vi "test Init Anaylsis Graph 1.vi"(11 "Test Case In":refnum<class "test Init Analysis Graph.lvclass">) -> (0 "error out":errorcluster, 3 "Test Case Out":refnum<class "test Init Analysis Graph.lvclass">)   [LabVIEW 2023, in "test Init Analysis Graph.lvclass"]
uses:
  test Init Analysis Graph.lvclass
  C:/Program Files/National Instruments/LabVIEW 2023/vi.lib/Astemes/LUnit/Test Case.lvclass
  source/Base Graph/Base Graph.lvclass/Base Graph.ctl
  source/Series Graph/Graph with Series View.lvclass/Graph with Series View.ctl
  source/Analysis Graph/Graph with Analysis Controls.lvclass/Graph with Analysis Controls.ctl
  <vilib>/Astemes/LUnit/Test Case.lvclass/Test Case.ctl
  source/Base Graph/Get Cursor Position.vi
  source/Series Graph/Get 1D Array Image Index and Length.vi
  source/Base Graph/Get Size.vi
  source/Series Graph/Get Shots.vi
  source/Analysis Graph/Update Z Cursors.vi
  <vilib>/Astemes/LUnit/Append Pass Result.vi
  <vilib>/Astemes/LUnit/Append Fail Result.vi
  source/Analysis Graph/Get Analysis ROI.vi
  source/Series Graph/Get Series Graph.vi
  <vilib>/Astemes/LUnit/Run In UI.vi
  source/Base Graph/Get ROI X-Y.vi
  <vilib>/Utility/error.llb/Clear Errors.vi
  source/Analysis Graph/Graph with Analysis Controls.lvclass
  D:/git/Lock-In-Thermography-Graphs/source/Series Graph/Graph with Series View.lvclass
  D:/git/Lock-In-Thermography-Graphs/source/Base Graph/Base Graph.lvclass
  source/Series Graph/Graph with Series View.lvclass
  <vilib>/Astemes/LUnit/Test Case.lvclass
  <vilib>/Analysis/NI_AALBase.lvlib
panel:
  in  "Z Range":cluster{"Index":u32, "Length":u32}={"Index"=0, "Length"=999}
  out "Signal Map Analysis":dbl[][](graph)
  out "Intensity Height Graph Analysis":cluster{"Array":dbl[], "Array":dbl[]}(graph)={"Array"=array[480 elements], "Array"=[0.0, 1.0, 2.0, 3.0, 4.0, 5.0, 6.0, 7.0, 8.0, 9.0, 10.0, 11.0, 12.0, 13.0, 14.0, 15.0, 16.0, 17.0, 18.0, 19.0, 20.0, 21.0, 22.0, 23.0, 24.0, 25.0, 26.0, 27.0, 28.0, 29.0, 30.0, 31.0, 32.0, 33.0, 34.0, 35.0, 36.0, 37.0, 38.0, 39.0, 40.0, 41.0, 42.0, 43.0, 44.0, 45.0, 46.0, 47.0, 48.0, 49.0, 50.0, 51.0, 52.0, 53.0, 54.0, 55.0, 56.0, 57.0, 58.0, 59.0, 60.0, 61.0, 62.0, 63.0, 64.0, 65.0, 66.0, 67.0, 68.0, 69.0, 70.0, 71.0, 72.0, 73.0, 74.0, 75.0, 76.0, 77.0, 78.0, 79.0, 80.0, 81.0, 82.0, 83.0, 84.0, 85.0, 86.0, 87.0, 88.0, 89.0, 90.0, 91.0, 92.0, 93.0, 94.0, 95.0, 96.0, 97.0, 98.0, 99.0, 100.0, 101.0, 102.0, 103.0, 104.0, 105.0, 106.0, 107.0, 108.0, 109.0, 110.0, 111.0, 112.0, 113.0, 114.0, 115.0, 116.0, 117.0, 118.0, 119.0, 120.0, 121.0, 122.0, 123.0, 124.0, 125.0, 126.0, 127.0, 128.0, 129.0, 130.0, 131.0, 132.0, 133.0, 134.0, 135.0, 136.0, 137.0, 138.0, 139.0, 140.0, 141.0, 142.0, 143.0, 144.0, 145.0, 146.0, 147.0, 148.0, 149.0, 150.0, 151.0, 152.0, 153.0, 154.0, 155.0, 156.0, 157.0, 158.0, 159.0, 160.0, 161.0, 162.0, 163.0, 164.0, 165.0, 166.0, 167.0, 168.0, 169.0, 170.0, 171.0, 172.0, 173.0, 174.0, 175.0, 176.0, 177.0, 178.0, 179.0, 180.0, 181.0, 182.0, 183.0, 184.0, 185.0, 186.0, 187.0, 188.0, 189.0, 190.0, 191.0, 192.0, 193.0, 194.0, 195.0, 196.0, 197.0, 198.0, 199.0, 200.0, 201.0, 202.0, 203.0, 204.0, 205.0, 206.0, 207.0, 208.0, 209.0, 210.0, 211.0, 212.0, 213.0, 214.0, 215.0, 216.0, 217.0, 218.0, 219.0, 220.0, 221.0, 222.0, 223.0, 224.0, 225.0, 226.0, 227.0, 228.0, 229.0, 230.0, 231.0, 232.0, 233.0, 234.0, 235.0, 236.0, 237.0, 238.0, 239.0, 240.0, 241.0, 242.0, 243.0, 244.0, 245.0, 246.0, 247.0, 248.0, 249.0, 250.0, 251.0, 252.0, 253.0, 254.0, 255.0, 256.0, 257.0, 258.0, 259.0, 260.0, 261.0, 262.0, 263.0, 264.0, 265.0, 266.0, 267.0, 268.0, 269.0, 270.0, 271.0, 272.0, 273.0, 274.0, 275.0, 276.0, 277.0, 278.0, 279.0, 280.0, 281.0, 282.0, 283.0, 284.0, 285.0, 286.0, 287.0, 288.0, 289.0, 290.0, 291.0, 292.0, 293.0, 294.0, 295.0, 296.0, 297.0, 298.0, 299.0, 300.0, 301.0, 302.0, 303.0, 304.0, 305.0, 306.0, 307.0, 308.0, 309.0, 310.0, 311.0, 312.0, 313.0, 314.0, 315.0, 316.0, 317.0, 318.0, 319.0, 320.0, 321.0, 322.0, 323.0, 324.0, 325.0, 326.0, 327.0, 328.0, 329.0, 330.0, 331.0, 332.0, 333.0, 334.0, 335.0, 336.0, 337.0, 338.0, 339.0, 340.0, 341.0, 342.0, 343.0, 344.0, 345.0, 346.0, 347.0, 348.0, 349.0, 350.0, 351.0, 352.0, 353.0, 354.0, 355.0, 356.0, 357.0, 358.0, 359.0, 360.0, 361.0, 362.0, 363.0, 364.0, 365.0, 366.0, 367.0, 368.0, 369.0, 370.0, 371.0, 372.0, 373.0, 374.0, 375.0, 376.0, 377.0, 378.0, 379.0, 380.0, 381.0, 382.0, 383.0, 384.0, 385.0, 386.0, 387.0, 388.0, 389.0, 390.0, 391.0, 392.0, 393.0, 394.0, 395.0, 396.0, 397.0, 398.0, 399.0, 400.0, 401.0, 402.0, 403.0, 404.0, 405.0, 406.0, 407.0, 408.0, 409.0, 410.0, 411.0, 412.0, 413.0, 414.0, 415.0, 416.0, 417.0, 418.0, 419.0, 420.0, 421.0, 422.0, 423.0, 424.0, 425.0, 426.0, 427.0, 428.0, 429.0, 430.0, 431.0, 432.0, 433.0, 434.0, 435.0, 436.0, 437.0, 438.0, 439.0, 440.0, 441.0, 442.0, 443.0, 444.0, 445.0, 446.0, 447.0, 448.0, 449.0, 450.0, 451.0, 452.0, 453.0, 454.0, 455.0, 456.0, 457.0, 458.0, 459.0, 460.0, 461.0, 462.0, 463.0, 464.0, 465.0, 466.0, 467.0, 468.0, 469.0, 470.0, 471.0, 472.0, 473.0, 474.0, 475.0, 476.0, 477.0, 478.0, 479.0]}
  out "Intensity Width Graph Analysis":cluster{"Array":dbl[], "Array":dbl[]}(graph)
  out "Z - Time Signal":u16[](graph)=[8685, 8675, 8685, 8678, 8689, 8675, 8659, 8679, 8685, 8681, 8681, 8682, 8675, 8687, 8678, 8679, 8686, 8681, 8671, 8674, 8685, 8680, 8679, 8667, 8687, 8682, 8683, 8675, 8675, 8677, 8683, 8679, 8685, 8686, 8687, 8679, 8688, 8683, 8679, 8683, 8681, 8685, 8684, 8677, 8677, 8680, 8677, 8674, 8697, 8693, 8683, 8704, 8687, 8692, 8700, 8688, 8691, 8687, 8699, 8697, 8693, 8710, 8707, 8709, 8693, 8711, 8690, 8699, 8699, 8710, 8709, 8700, 8712, 8701, 8714, 8718, 8710, 8723, 8717, 8718, 8727, 8731, 8715, 8724, 8729, 8735, 8725, 8745, 8724, 8730, 8746, 8744, 8740, 8729, 8737, 8722, 8748, 8727, 8736, 8747, 8746, 8742, 8739, 8752, 8746, 8745, 8748, 8748, 8738, 8737, 8737, 8747, 8770, 8768, 8766, 8763, 8774, 8769, 8761, 8753, 8758, 8747, 8766, 8775, 8780, 8771, 8775, 8785, 8766, 8778, 8762, 8772, 8783, 8785, 8778, 8778, 8787, 8796, 8807, 8798, 8789, 8792, 8804, 8799, 8794, 8799, 8796, 8805, 8789, 8792, 8805, 8813, 8805, 8796, 8805, 8798, 8812, 8816, 8811, 8809, 8821, 8821, 8808, 8804, 8818, 8822, 8826, 8829, 8810, 8834, 8808, 8820, 8814, 8821, 8822, 8825, 8825, 8830, 8836, 8821, 8842, 8826, 8819, 8820, 8841, 8827, 8833, 8838, 8835, 8842, 8830, 8839, 8829, 8831, 8839, 8849, 8838, 8842, 8836, 8844, 8832, 8845, 8841, 8857, 8858, 8844, 8836, 8839, 8828, 8856, 8843, 8854, 8851, 8852, 8837, 8827, 8848, 8864, 8846, 8839, 8840, 8851, 8840, 8846, 8861, 8838, 8849, 8857, 8854, 8847, 8862, 8844, 8854, 8857, 8857, 8858, 8850, 8843, 8851, 8861, 8845, 8851, 8841, 8841, 8853, 8855, 8857, 8847, 8855, 8838, 8844, 8847, 8847, 8849, 8841, 8854, 8855, 8857, 8845, 8855, 8848, 8865, 8845, 8846, 8834, 8845, 8861, 8860, 8860, 8847, 8852, 8849, 8847, 8862, 8853, 8854, 8857, 8870, 8846, 8848, 8848, 8859, 8851, 8847, 8839, 8851, 8847, 8849, 8862, 8847, 8841, 8846, 8859, 8847, 8854, 8861, 8846, 8861, 8848, 8865, 8858, 8868, 8850, 8860, 8858, 8869, 8863, 8866, 8855, 8865, 8870, 8857, 8867, 8851, 8869, 8861, 8866, 8862, 8867, 8883, 8873, 8869, 8881, 8880, 8875, 8882, 8876, 8876, 8885, 8883, 8875, 8879, 8890, 8883, 8876, 8878, 8887, 8878, 8878, 8890, 8896, 8885, 8885, 8890, 8892, 8902, 8887, 8901, 8893, 8892, 8885, 8892, 8904, 8901, 8904, 8908, 8908, 8903, 8906, 8906, 8921, 8904, 8905, 8911, 8929, 8925, 8921, 8935, 8934, 8914, 8925, 8919, 8931, 8925, 8927, 8918, 8933, 8942, 8956, 8920, 8950, 8946, 8952, 8954, 8946, 8937, 8935, 8944, 8942, 8950, 8951, 8949, 8957, 8964, 8950, 8963, 8959, 8953, 8948, 8955, 8969, 8965, 8968, 8972, 8973, 8976, 8983, 8973, 8969, 8981, 8977, 8977, 8967, 8978, 8979, 8993, 8983, 8985, 8984, 8972, 8989, 8986, 8984, 8986, 8987, 8991, 8991, 8989, 8992, 8996, 8993, 8991, 8991, 9001, 8984, 8992, 8989, 8986, 9001, 8988, 8978, 8994, 9006, 9000, 9007, 8990, 8993, 9009, 9011, 9003, 8999, 9004, 8994, 9007, 8998, 9000, 8999, 8995, 9000, 8999, 9004, 9012, 8997, 8995, 9001, 8995, 9004, 8995, 9010, 8997, 8989, 8995, 9007, 9006, 9002, 9002, 9002, 8998, 8983, 9018, 8991, 8996, 9005, 9002, 8987, 8998, 9000, 8991, 9003, 8995, 9005, 8994, 8999, 9000, 8989, 8990, 8991, 8998, 8991, 9001, 8999, 8996, 8997, 8993, 8998, 8993, 9008, 8996, 8991, 9001, 9013, 8992, 9006, 8998, 8999, 8995, 9005, 8993, 8999, 9002, 8999, 9007, 8996, 8996, 8997, 9009, 9004, 9001, 8999, 8977, 9008, 9009, 9005, 8994, 9003, 8992, 8995, 9012, 9008, 9009, 8999, 8998, 8988, 9010, 8988, 8990, 9006, 8999, 8984, 8983, 9003, 8993, 9004, 9008, 9010, 8981, 9002, 8994, 8994, 8994, 9009, 9020, 9012, 9016, 9004, 9018, 9022, 9015, 9013, 9008, 9017, 9019, 9005, 9013, 9023, 9014, 9029, 9021, 9010, 9020, 9027, 9018, 9021, 9032, 9007, 9029, 9022, 9010, 9018, 9024, 9025, 9035, 9029, 9026, 9036, 9022, 9040, 9042, 9041, 9024, 9041, 9046, 9049, 9044, 9048, 9036, 9047, 9055, 9053, 9050, 9056, 9047, 9061, 9056, 9045, 9056, 9064, 9056, 9058, 9082, 9055, 9062, 9064, 9065, 9068, 9062, 9048, 9049, 9054, 9070, 9064, 9066, 9088, 9071, 9084, 9075, 9075, 9082, 9075, 9076, 9083, 9083, 9098, 9092, 9100, 9078, 9093, 9094, 9085, 9099, 9103, 9084, 9091, 9088, 9102, 9106, 9102, 9101, 9083, 9097, 9098, 9097, 9104, 9102, 9113, 9100, 9100, 9106, 9112, 9106, 9111, 9107, 9102, 9104, 9110, 9124, 9112, 9118, 9114, 9115, 9114, 9115, 9133, 9125, 9120, 9111, 9118, 9118, 9131, 9115, 9121, 9126, 9120, 9120, 9126, 9125, 9125, 9128, 9117, 9135, 9126, 9128, 9134, 9121, 9119, 9114, 9133, 9124, 9124, 9124, 9136, 9124, 9133, 9128, 9123, 9134, 9134, 9135, 9135, 9126, 9120, 9139, 9133, 9145, 9129, 9123, 9127, 9137, 9136, 9133, 9123, 9129, 9128, 9127, 9145, 9115, 9129, 9130, 9124, 9127, 9115, 9120, 9115, 9119, 9113, 9127, 9126, 9119, 9113, 9125, 9123, 9115, 9120, 9119, 9121, 9119, 9128, 9123, 9126, 9121, 9118, 9111, 9113, 9120, 9106, 9122, 9130, 9107, 9111, 9100, 9115, 9107, 9124, 9119, 9132, 9110, 9106, 9126, 9119, 9102, 9111, 9102, 9100, 9119, 9116, 9136, 9119, 9120, 9106, 9132, 9119, 9125, 9107, 9119, 9126, 9127, 9122, 9123, 9129, 9121, 9129, 9117, 9118, 9114, 9122, 9119, 9127, 9126, 9124, 9124, 9121, 9131, 9122, 9123, 9122, 9141, 9133, 9135, 9127, 9129, 9136, 9138, 9137, 9111, 9134, 9134, 9134, 9139, 9138, 9138, 9117, 9133, 9141, 9135, 9132, 9142, 9137, 9155, 9143, 9150, 9155, 9147, 9149, 9154, 9163, 9143, 9150, 9154, 9147, 9156, 9150, 9162, 9160, 9159, 9154, 9166, 9161, 9170, 9162, 9159, 9171, 9168, 9175, 9175, 9158, 9173, 9179, 9164, 9185, 9163, 9172, 9188, 9181, 9190, 9185, 9181, 9179, 9192, 9182, 9189, 9179, 9187, 9202, 9198, 9182, 9174, 9180, 9186, 9202, 9202, 9199, 9202, 9213, 9206, 9208, 9188, 9200, 9213, 9211, 9206, 9198, 9203, 9200, 9217, 9202, 9212, 9217, 9211, 9221, 9229, 9226, 9226, 9212, 9224, 9210, 9213, 9216, 9226, 9228, 9205, 9214, 9226, 9230, 9236, 9233, 9218, 9243, 9238, 9242, 9224, 9239, 9238, 9238, 9242, 9231, 9244, 9224, 9239, 9232, 9244, 9242, 9241, 9231, 9240, 9231, 9245, 9239, 9238, 9231, 9239, 9231, 9238, 9249, 9245, 9233, 9238, 9247, 9247, 9246, 9243, 9249, 9248, 9238, 9247, 9250, 9231, 9232, 9244, 9243, 9237, 9241, 9240, 9234, 9244, 9244, 9257, 9246, 9240, 9237, 9236, 9241, 9255, 9236, 9247, 9240, 9245, 9239, 9237, 9224, 9234, 9233, 9238, 9234, 9237, 9238, 9237, 9225, 9236, 9244, 9219]
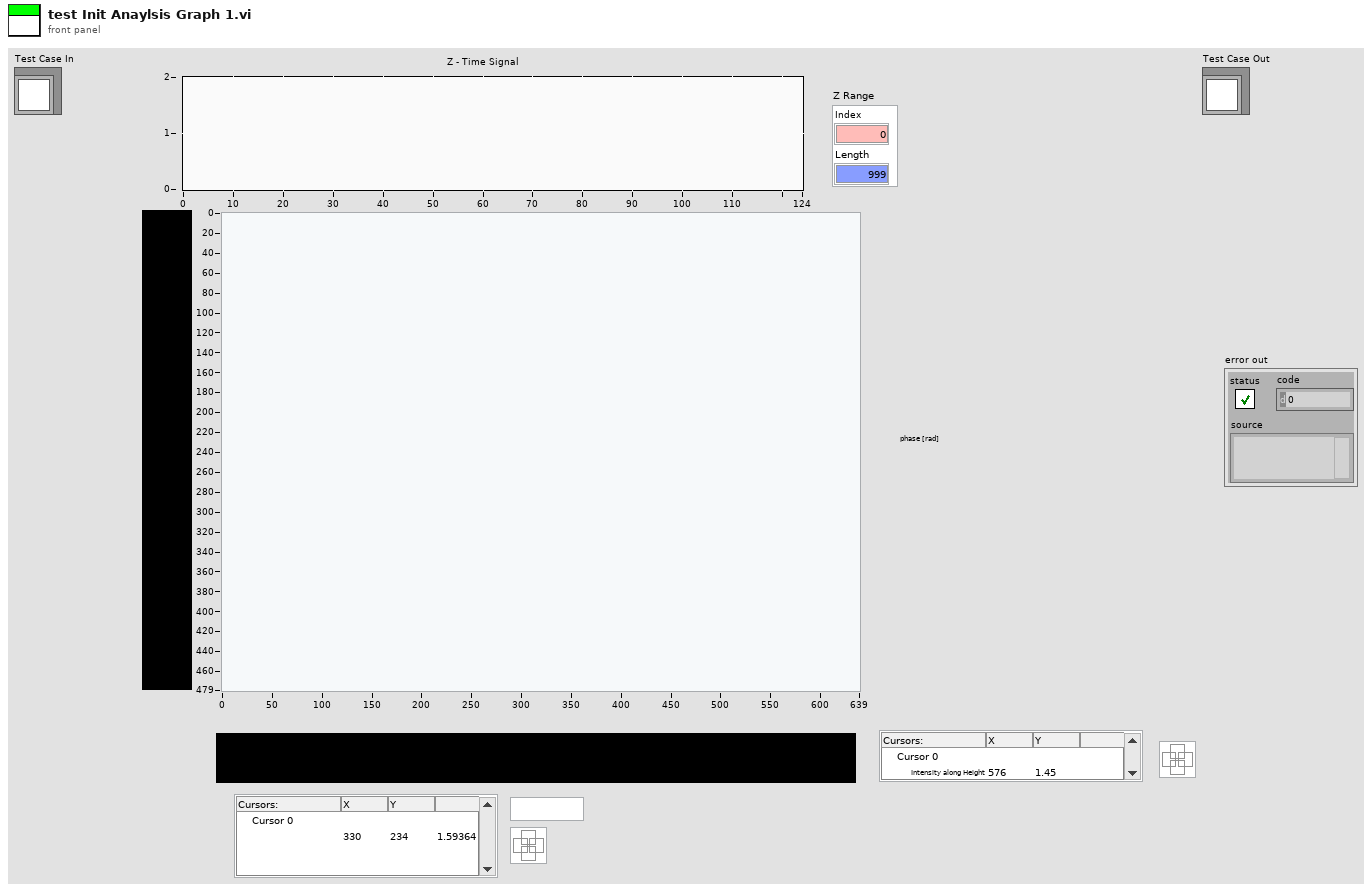
[diagram p1: front panel]
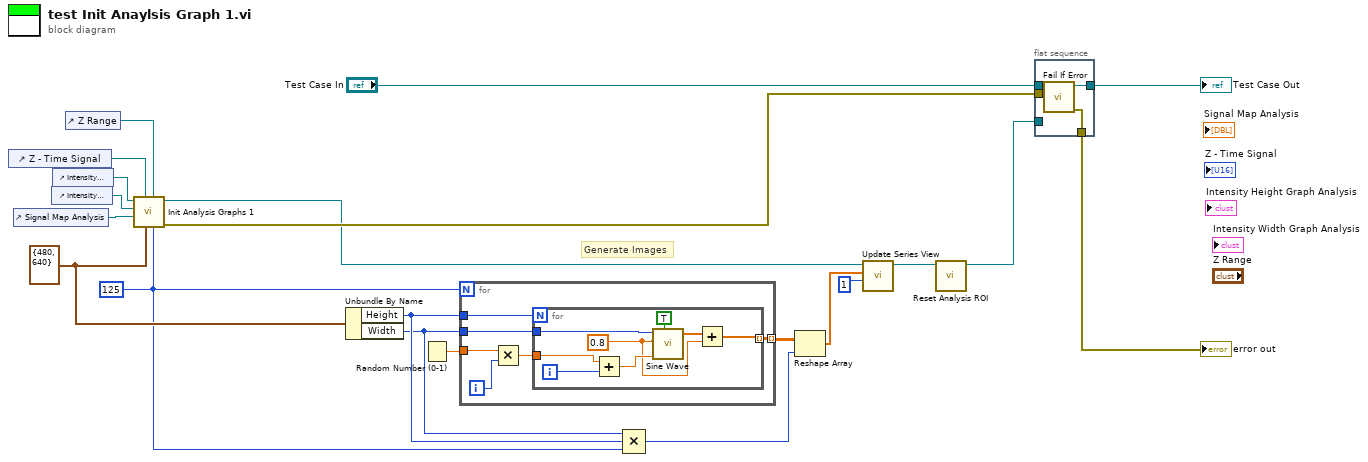
[diagram p0: block diagram]
diagram:
  w4 = u32 125 ("Shots")
  w5 = cluster{"Height":u32, "Width":u32} {"Height"=480, "Width"=640} ("Image Size")
  # "Generate Images"
  n1 = control-ref of="Z - Time Signal"() -> (w13:refnum<vi>)
  n2 = control-ref of="Signal Map Analysis"() -> (w14:refnum<vi>)
  n3 = control-ref of="Intensity Width Graph Analysis"() -> (w15:refnum<vi>)
  n4 = control-ref of="Intensity Height Graph Analysis"() -> (w16:refnum<vi>)
  n5 = control-ref of="Z Range"() -> (w17:refnum<vi>)
  n6 = call "Init Analysis Graphs 1.vi"("Shots"=w4, "Z Range"=w17, "Image Size"=w5, "Z - Time Signal"=w13, "Signal Map Analysis"=w14, "Intensity Width Graph Analysis"=w15, "Intensity Height Graph Analysis"=w16) -> ("error out"=w18:errorcluster, "Analysis Graph out"=w3:refnum<class "Graph with Analysis Controls.lvclass">)  [unwired: 3 in]
  n7 = Unbundle By Name(w5) -> ("Height"=w12:u32, "Width"=w11:u32)
  n8 = Random Number (0-1)() -> (number: 0 to 1=w6:dbl)
  n9 = for {
    N: w4 -> [_]
    tunnel: [w27] -> w7 mode=indexing
    tunnel: w11 -> [w26]
    tunnel: w12 -> [w25]
    tunnel: w6 -> [w22]
    i -> [w24]
    n10 = Multiply(x=w22, y=w24) -> (x*y=w23:dbl)
    n11 = for {
      N: w25 -> [_]
      tunnel: [w29] -> w27 mode=indexing
      tunnel: w26 -> [w32]
      tunnel: w23 -> [w31]
      i -> [w34]
      w28 = 0.8
      n12 = Add(x=w31, y=w34) -> (x+y=w33:dbl)
      n13 = call <vilib>:"Sine Wave.vi"("samples"=w32, "amplitude"=w28, "phase in"=w33, "reset phase"=TRUE) -> ("sine wave"=w30:dbl[])  [unwired: 1 in, 2 out]
      n14 = Add(x=w30, y=w28) -> (x+y=w29:dbl[])
    }
  }
  n15 = Compound Arithmetic op=MULTIPLY(w11, w12, w4) -> (w10:u32)
  n16 = Reshape Array(w7, w10) -> (w9:dbl[])
  n17 = call "Update Series View.vi"("Image #"=u32 1, "Image Series"=w9, "Series Graph in"=w3) -> ("Series Graph out"=w2:refnum<class "Graph with Analysis Controls.lvclass">)  [unwired: 8 in]
  n18 = call "Reset Analysis ROI.vi"("Analysis Graph in"=w2) -> ("Analysis Graph out"=w1:refnum<class "Graph with Analysis Controls.lvclass">)  [unwired: 10 in]
  n19 = flat-sequence {
    tunnel: "Test Case In" -> [w39]
    tunnel: [w38] -> w20
    tunnel: [w37] -> w19
    tunnel: w18 -> [w36]
    tunnel: w1 -> [_]
    frame #0 {
      n20 = call <vilib>:"Fail If Error.vi"("Assert error"=w36, "LUnit Test Case In"=w39) -> ("error out"=w37:errorcluster, "LUnit Test Case Out"=w38:refnum<class "test Init Analysis Graph.lvclass">)  [unwired: 8 in]
    }
  }
  "error out" <- w19
  "Test Case Out" <- w20
